vi "Kxx_Kxy_B_cs580_KEguard.vi"() -> ()   [LabVIEW 2023]
uses:
  Z:/Labview Control Software/Kxx_Kxy_B_cs580_v3_LV20/Z/Labview Control Software/Keithley 622x LV 2009/Utility/Typedefs/KE622x -- Instrument Type.ctl
  Typedefs/Kxx_Kxy_state_machine_cases.ctl
  Z:/Labview Control Software/Keithley 622x LV 2009/Typedefs/KE622x -- On Off Control.ctl
  Z:/Labview Control Software/Keithley 622x LV 2009/Configure/Output/Typedefs/KE6221 -- Output Response.ctl
  Z:/Labview Control Software/Keithley 622x LV 2009/Configure/Source/Typedefs/KE622x -- Voltage Limit.ctl
  <vilib>/Analysis/1siggen.llb/Ramp Pattern by Samples.vi
  <vilib>/Analysis/baseanly.llb/Mean (DBL).vi
  <vilib>/Instr/_visa.llb/VISA Configure Serial Port (Instr).vi
  <vilib>/Utility/file.llb/Read Delimited Spreadsheet (DBL).vi
  Global Variables/MQM Data Transfer All.vi
  <vilib>/Analysis/1siggen.llb/Ramp Pattern by Delta.vi
  <vilib>/Utility/file.llb/Write To Spreadsheet File (string).vi
  <instrlib>/Keithley 622x LV 2009/Keithley 622x.lvlib
  <vilib>/Analysis/NI_AALBase.lvlib
  Drivers/Keithley 2182/Keithley 2182.lvlib
  <vilib>/Analysis/NI_AALPro.lvlib
panel:
  out "error out":errorcluster
  in  "Kxy data":dbl[](array[numeric])
  in  "Kxx data":dbl[](array[numeric])
  in  "T_avg data":dbl[](array[numeric])
  in  "dTxx":dbl
  in  "HTR Power":dbl
  in  "dTxy":dbl
  in  "T_avg":dbl
  in  "T_H Array":dbl[](array[numeric])
  in  "T_C1 Array":dbl[](array[numeric])
  in  "T_C2 Array":dbl[](array[numeric])
  in  "HTR Voltage Array":dbl[](array[numeric])
  in  "?":enum32{"Setup", "Plotting", "Error Readouts"}(tab)
  in  "DeltaT (fraction of tsp)":dbl=0.05
  in  "Sample_t":dbl
  in  "Sample_w":dbl
  in  "Sample_Lxx":dbl
  in  "Heater Current File (H, T, current)":path
  out "Heater Current \nArray":dbl[](array[numeric])
  out "Ramp Pattern":dbl[](array[numeric])
  in  "Tstart (K)":dbl=3.0
  in  "Tend (K)":dbl=4.0
  in  "Steps":i16=2
  in  "Log (on)\nLin (off) (Temperature setpoints)":bool=TRUE
  in  "Initial Heater Current (A)":dbl=1e-06
  in  "Hstart (Oe)":dbl
  in  "Hend (Oe)":dbl
  in  "Field Steps":i16=1
  in  "Log (on)\nLin (off)  (Field setpoints)":bool
  in  "T_H Lockin":enum16{"LI1", "LI2", "LI3"}(ring)
  in  "T_C1 Lockin":enum16{"LI1", "LI2", "LI3"}(ring)=enum."LI2"
  in  "T_C2 Lockin":enum16{"LI1", "LI2", "LI3"}(ring)=enum."LI3"
  in  "Sample_Lxy":dbl=0.0005
  in  "Test?":bool
  in  "Calibration Only?":bool
  in  "Exchange gas?":bool
  in  "Preset Heater Current Array?":bool
  in  "T Current Source":refnum<visa-resource-name>="6221B"
  in  "HTR Current Source":refnum<visa-resource-name>="CS580-1"
  in  "DC Voltmeter":refnum<visa-resource-name>="2182"
  in  "Thermometer Frequency (Hz)":string="37"
  in  "Initial Thermometer Current (A)":string="1.4142e-7"
  in  "Final Field (Oe)":dbl
  in  "Final Temperature (K)":dbl=1.7
  in  "R_H coeffs file":path
  in  "R_C1 coeffs file":path
  in  "R_C2 coeffs file":path
  in  "R_C1 domain file":path
  in  "R_C2 domain file":path
  in  "R_H domain file":path
  in  "Field selection":u16(ring) items=["0.000000"]
  out "Calibration confirmed":bool
  out "R_C1 coeffs":dbl[](array[numeric])
  out "R_C2 coeffs":dbl[](array[numeric])
  out "R_H coeffs":dbl[](array[numeric])
  out "R_C1 Log Domain":dbl[](array[numeric])
  out "R_C2 Log Domain":dbl[](array[numeric])
  out "R_H Log Domain":dbl[](array[numeric])
  in  "Confirm Calibration":bool
  in  "Filename":path=path "C:/User Data/Luke/Kxx/NaYSe2/NaYSe2_1p7_100K_log_100_9T_8_23_21"
  in  "Heater Only?":bool
  in  "DC Keithley":refnum<visa-resource-name>
  out "Kxx Plot":cluster{dbl[], dbl[]}(graph)
  out "Kxy Plot":cluster{dbl[], dbl[]}(graph)
  out "All Data":cluster{dbl[], dbl[]}[](graph)
  in  "Finish":bool
  out "Data Rate (ms)":u32
  in  "Delay (ms)":dbl=300.0
  in  "Quick Data Recording":bool=TRUE
  out "Tsp":dbl
  out "HTR_Current":dbl
  out "Mask":dbl
  out "HTR_Voltage":dbl
  out "T_H":dbl
  out "T_C1":dbl
  out "I_therm":dbl
  out "T_C2":dbl
  in  "Display Elements":cluster{"X":bool, "Y":bool, "Name":u16}[](array[cluster]) {"Name" items=["Time (ms)", "Temperature (K)", "Field (T)", "LI_1_X", "LI_1_theta", "LI_3_X", "LI_3_theta", "LI_2_X", "LI_2_theta", "DC_V", "DC_I", "mask", "tsp", "I_therm", "T_H", "T_C1", "T_C2", "Fieldsp"]}
  in  "X-Axis":u16(ring) items=["Linear", "Reciprocal", "Log10"]
  in  "Y-Axis":u16(ring) items=["Linear", "Reciprocal", "Log10"]
  out "Fieldsp":dbl
  out "Global Stop":bool
  out "QD error out":errorcluster
  out "KE6221 error out":errorcluster
  out "KE2182 error out":errorcluster
  # "TURN ON HIGH VACUUM!"
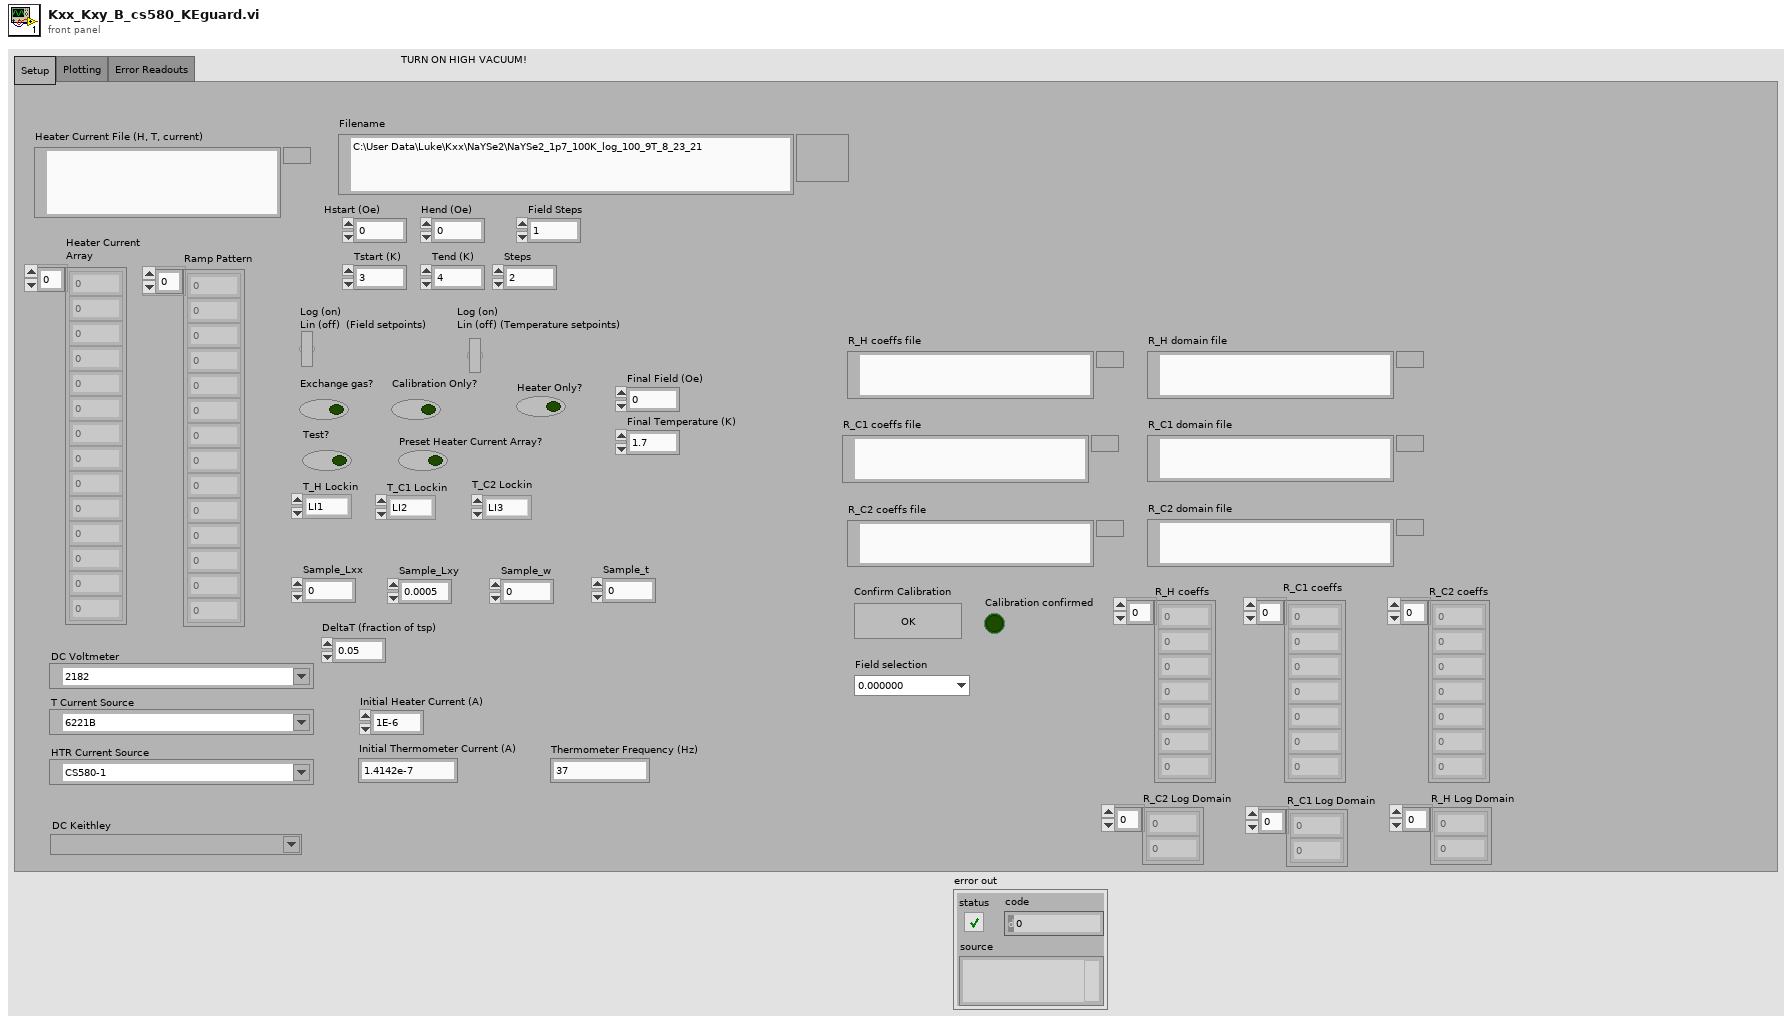
[diagram p1: front panel]
types:
  T1 = typedef "Keithley 622x.lvlib/KE622x -- Instrument Type.ctl" = enum16{"KE6220", "KE6221"}
  T2 = typedef "Kxx_Kxy_state_machine_cases.ctl" = enum16{"Initialize", "Wait to Stabilize (no heat)", "Measure (no heat)", "Turn on Heater, stabilize", "Measure (heat)", "Turn off Heater", "Assign Heater Current", "Plot Kxx, Kxy", "End"}
  T3 = typedef "Keithley 622x.lvlib/KE622x -- Voltage Limit.ctl" = dbl
  T4 = typedef "Keithley 622x.lvlib/KE6221 -- Output Response.ctl" = enum16{"Fast", "Slow"}
  T5 = typedef "Keithley 622x.lvlib/KE622x -- On Off Control.ctl" = enum16{"Off", "On"}
  T6 = cluster{"T_avg data":dbl[], "Kxx data":dbl[], "Kxy data":dbl[]}
  T7 = cluster{"T_avg":dbl, "dTxx":dbl, "dTxy":dbl, "HTR Power":dbl, "HTR Voltage Array":dbl[], "T_H Array":dbl[], "T_C1 Array":dbl[], "T_C2 Array":dbl[], "error out":errorcluster}
  T8 = typedef "ZI_Frontpanel_All.ctl" = cluster{"Lockin 1 Demod 0":cluster{"R(V)":dbl, "Theta (deg)":dbl, "Timestamp (ms)":u32, "X(V)":dbl, "Y(V)":dbl, "frequency (Hz)":dbl, "output voltage (V)":dbl}, "Lockin 2 Demod 0":cluster{"R(V)":dbl, "Theta (deg)":dbl, "Timestamp (ms)":u32, "X(V)":dbl, "Y(V)":dbl, "frequency (Hz)":dbl, "output voltage (V)":dbl}, "Lockin 3 Demod 0":cluster{"R(V)":dbl, "Theta (deg)":dbl, "Timestamp (ms)":u32, "X(V)":dbl, "Y(V)":dbl, "frequency (Hz)":dbl, "output voltage (V)":dbl}, "Lockin 4 Demod 0":cluster{"R(V)":dbl, "Theta (deg)":dbl, "Timestamp (ms)":u32, "X(V)":dbl, "Y(V)":dbl, "frequency (Hz)":dbl, "output voltage (V)":dbl}, "LI1 active":bool, "LI2 active":bool, "LI3 active":bool, "LI4 active":bool}
  T9 = typedef "PPMS_Status.ctl" = cluster{"Field":cluster{"Field (T)":dbl, "Field stable":bool, "Timestamp (ms)":u32}, "Temperature":cluster{"Temperature (K)":dbl, "Temperature stable":bool, "Timestamp (ms)":u32}}
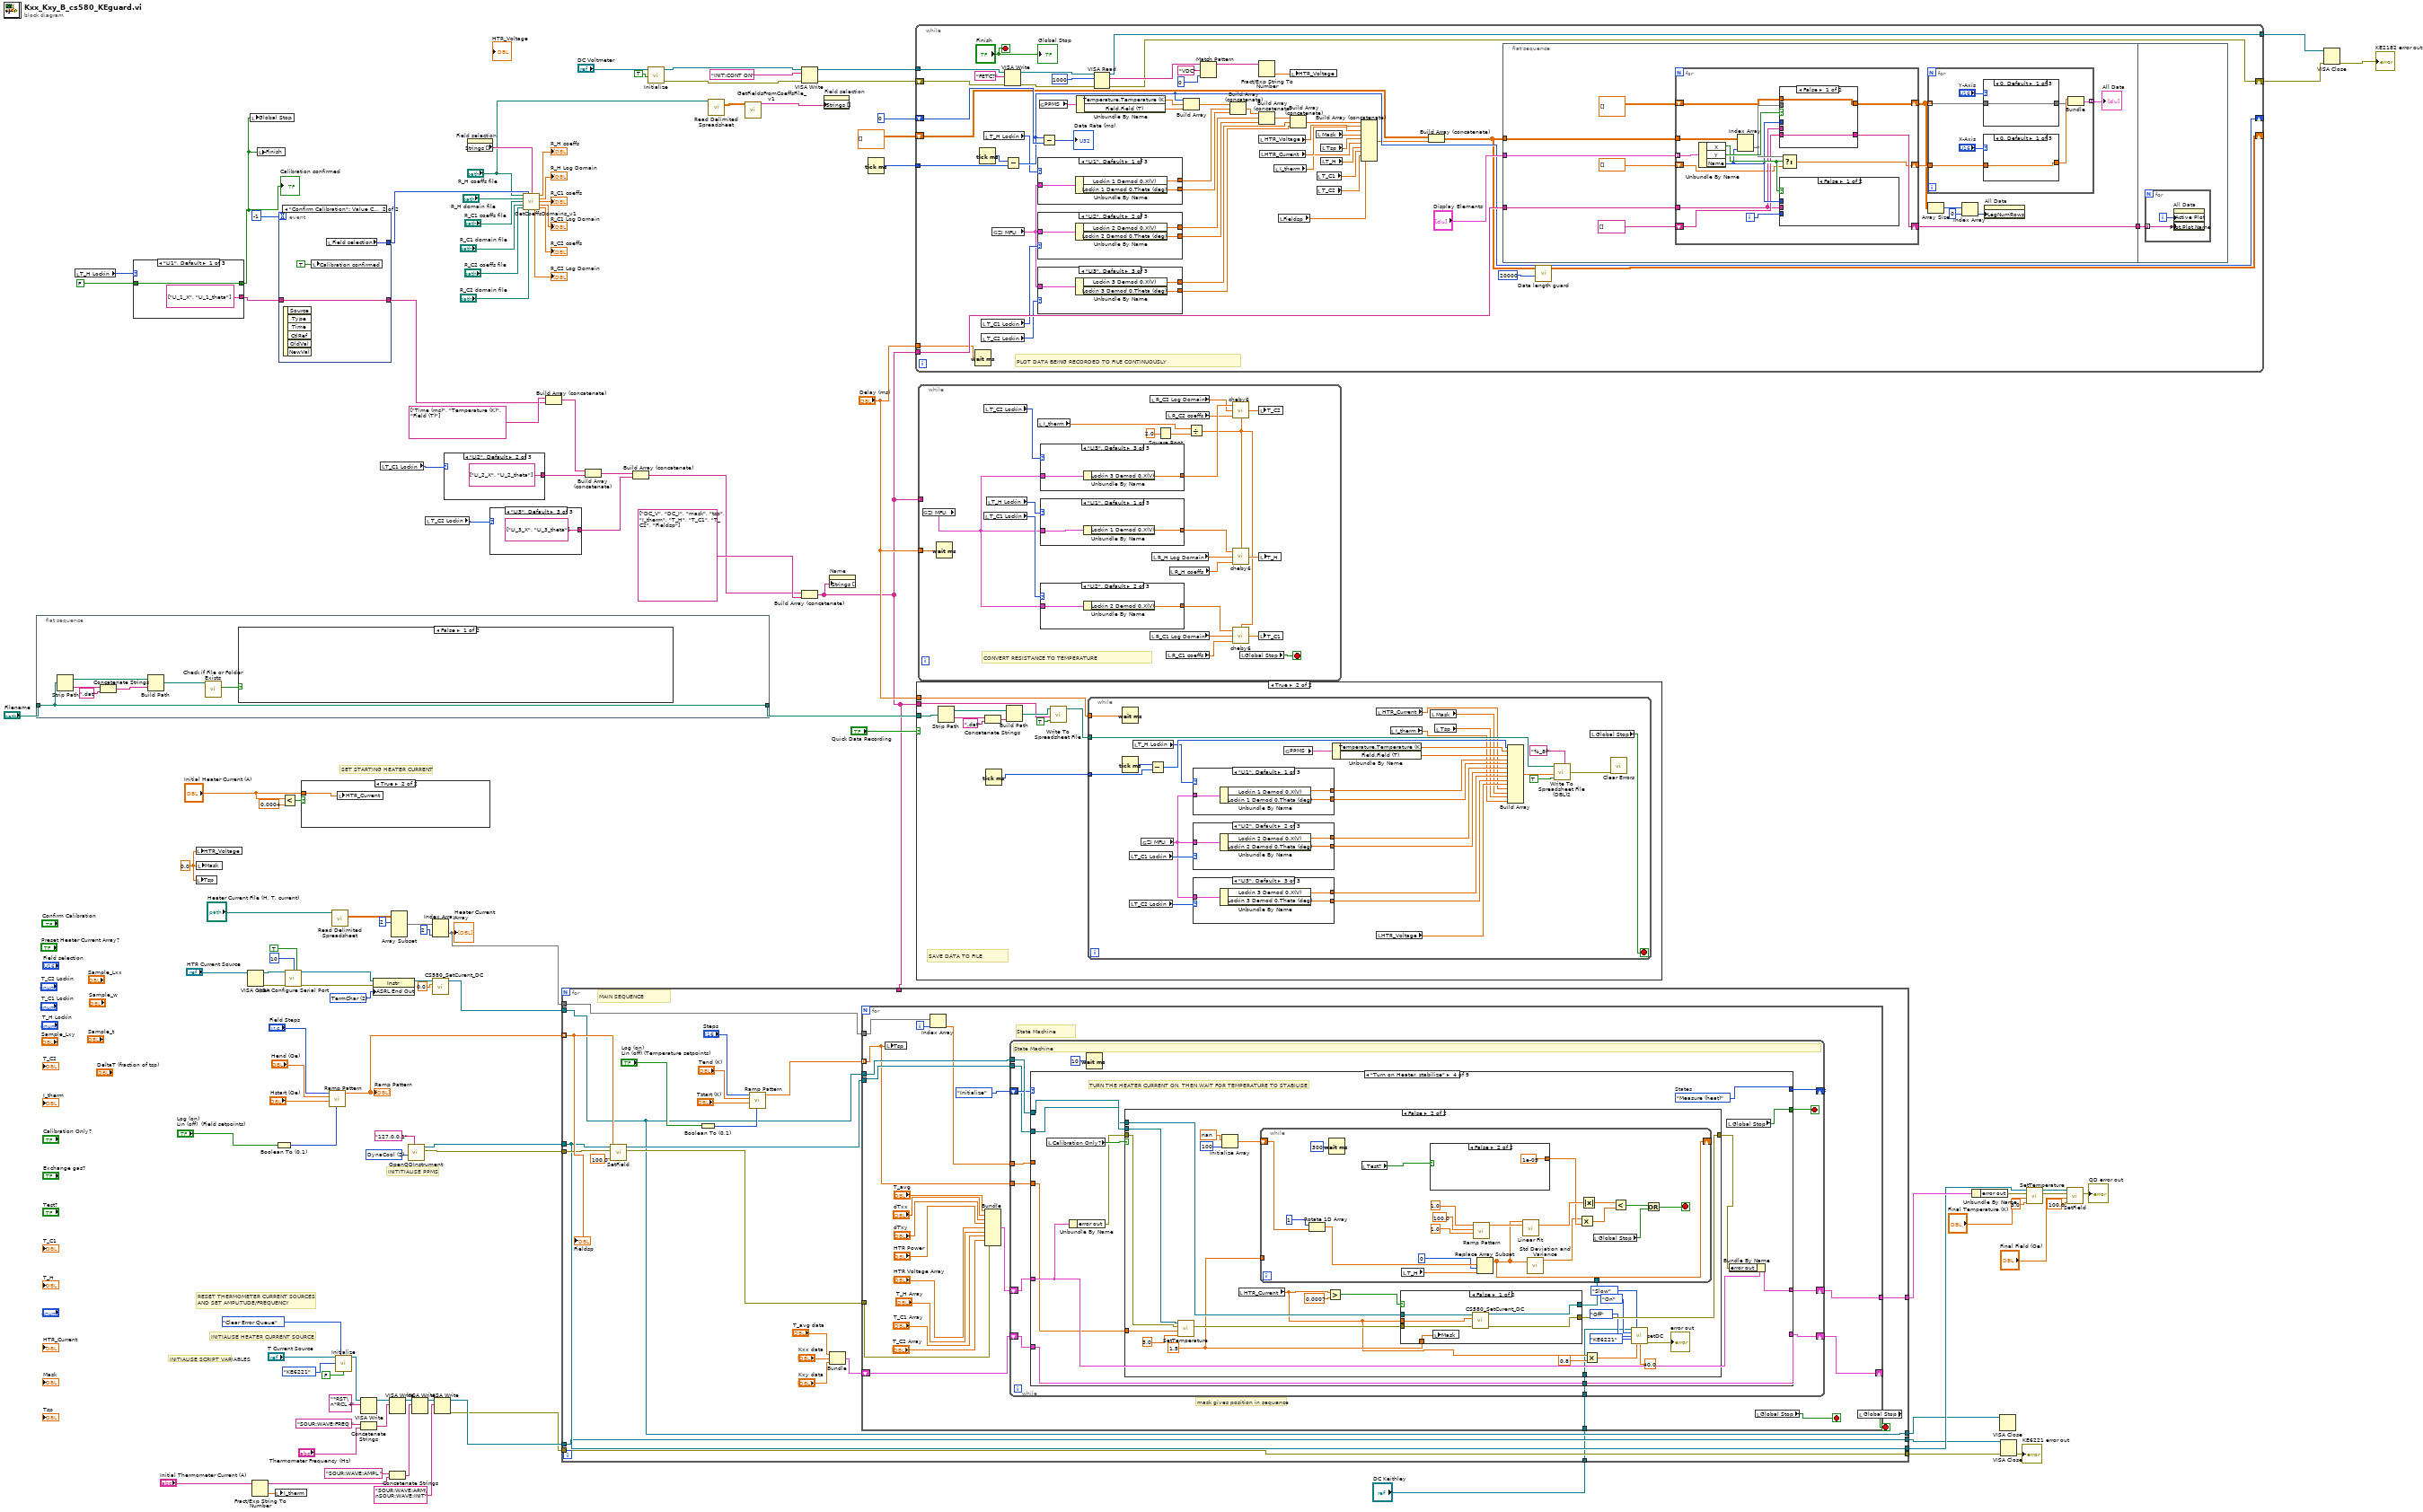
[diagram p0: block diagram]
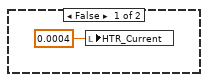
[diagram p2: hidden frame]
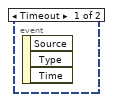
[diagram p3: hidden frame]
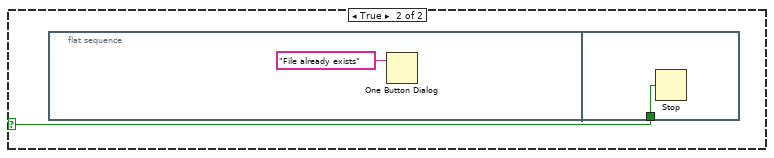
[diagram p4: hidden frame]
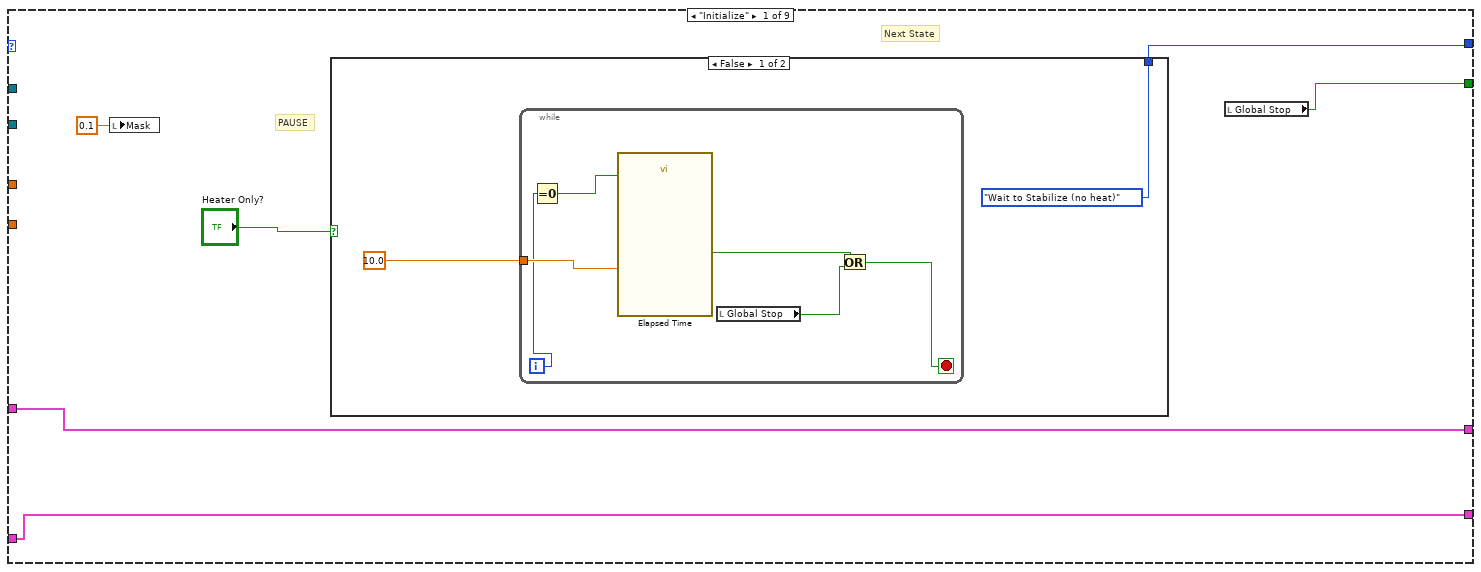
[diagram p5: hidden frame]
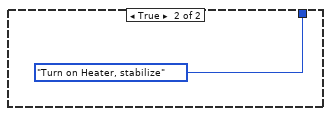
[diagram p6: hidden frame]
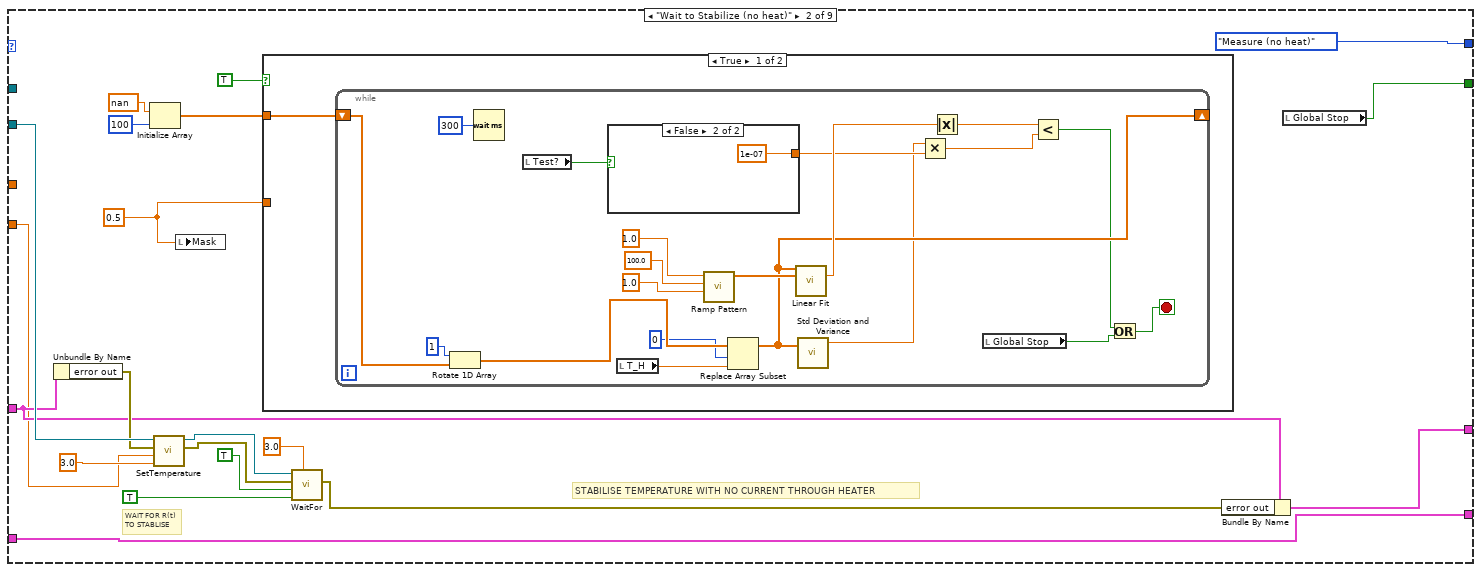
[diagram p7: hidden frame]
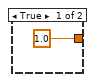
[diagram p8: hidden frame]
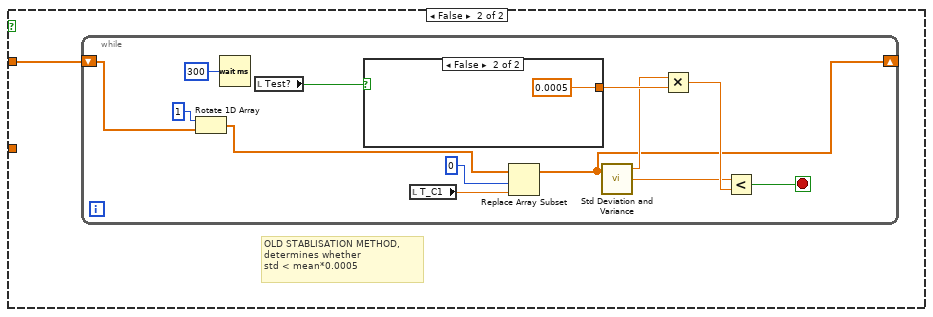
[diagram p9: hidden frame]
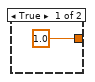
[diagram p10: hidden frame]
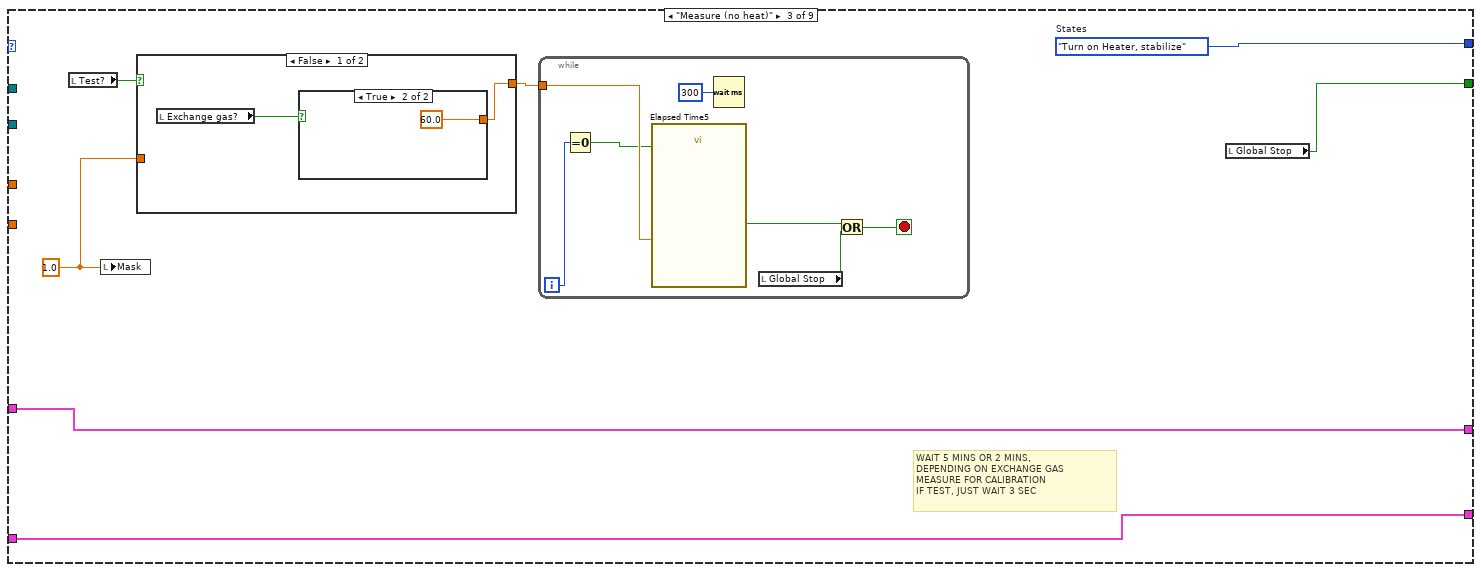
[diagram p11: hidden frame]
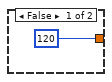
[diagram p12: hidden frame]
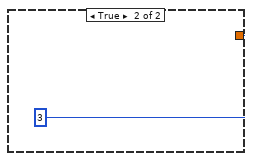
[diagram p13: hidden frame]
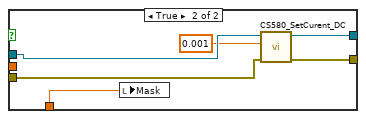
[diagram p15: hidden frame]
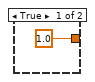
[diagram p16: hidden frame]
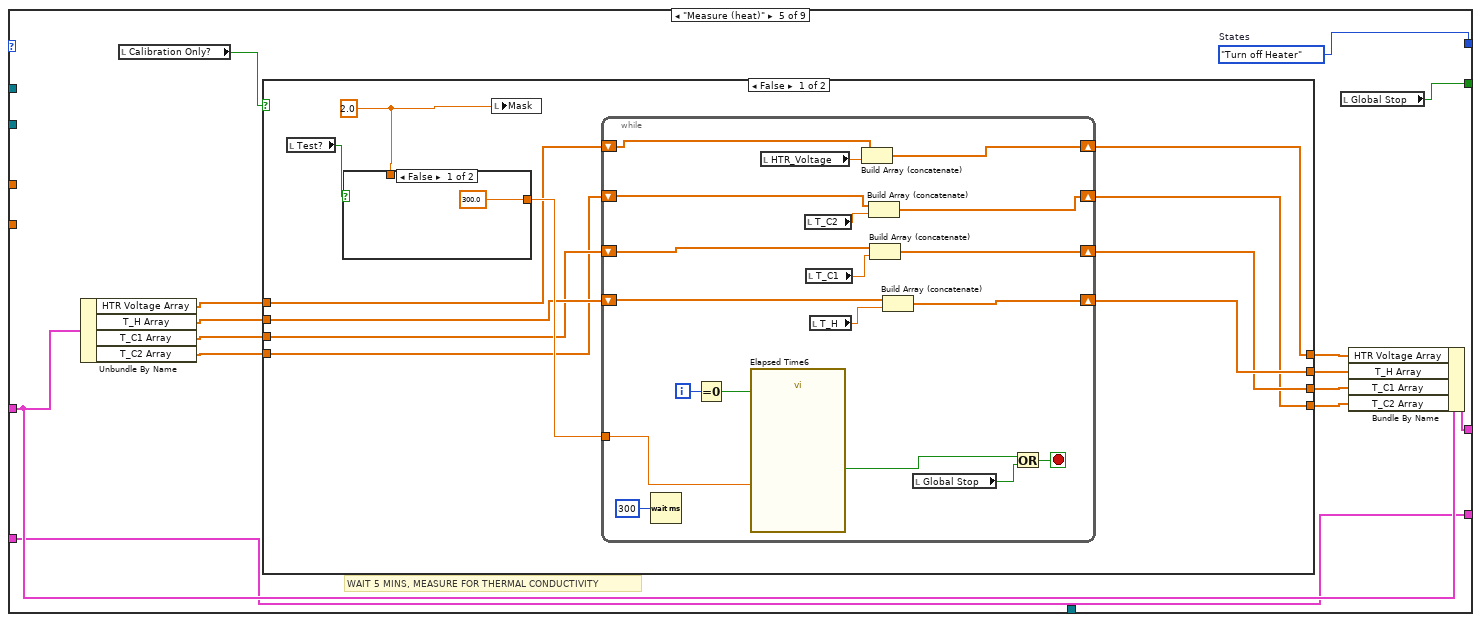
[diagram p17: hidden frame]
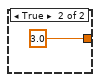
[diagram p18: hidden frame]
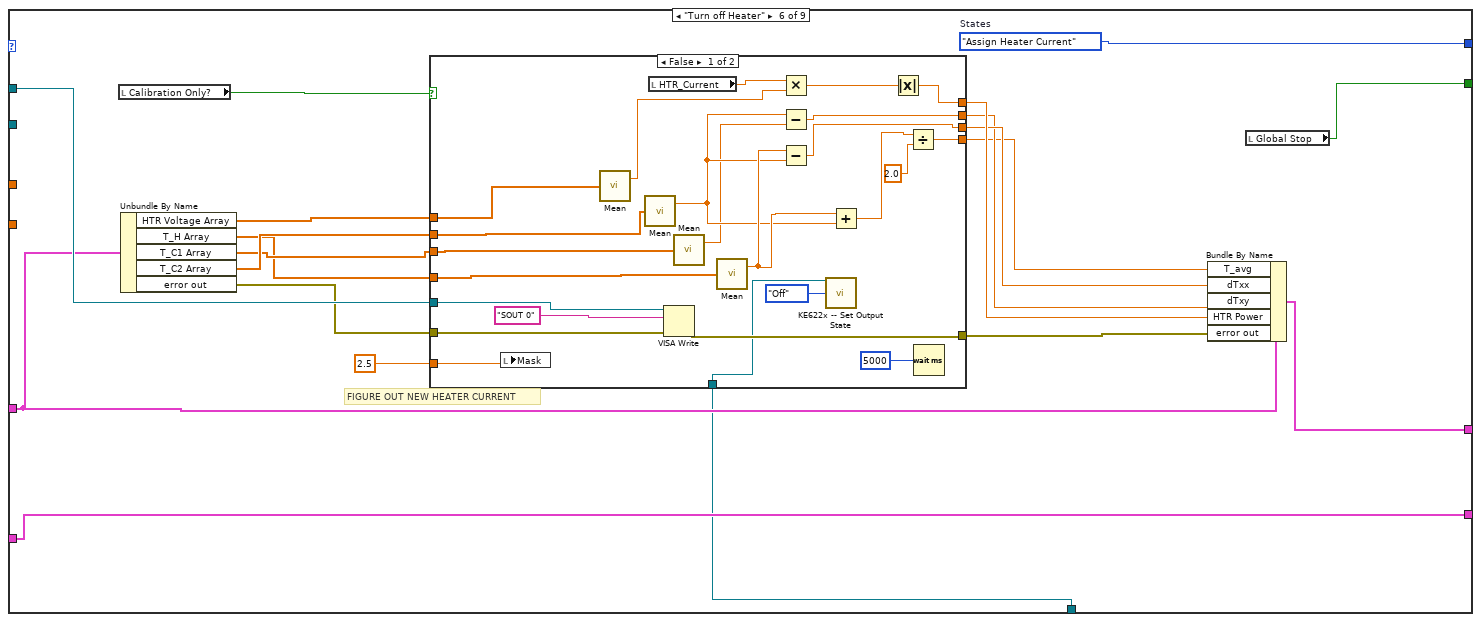
[diagram p20: hidden frame]
diagram:
  w85 = u16 2 items=["None", "Last Bit", "TermChar", "Break"] ("Serial Settings:End Mode for Writes")
  w103 = 0.0 ("Mask")
  w110 = 2 items=["PPMS", "VersaLab", "DynaCool", "SVSM"] ("Instrument Type")
  # "SET STARTING HEATER CURRENT"
  # "INITIALISE HEATER CURRENT SOURCE"
  # "RESET THERMOMETER CURRENT SOURCES\nAND SET AMPLITUDE/FREQUENCY"
  # "INITITIALISE PPMS"
  # "INITIALISE SCRIPT VARIABLES"
  n1 = flat-sequence {
    tunnel: "Filename" -> [w117]
    tunnel: [w117] -> w37
    frame #0 {
      n2 = Strip Path(path=w117) -> (stripped path=w121:path, name=w118:string)
      n3 = Concatenate Strings(w118, ".dat") -> (w120:string)
      n4 = Build Path(base path=w121, name or relative path=w120) -> (appended path=w116:path)
      n5 = call <vilib>:"Check if File or Folder Exists.vi"("path"=w116) -> ("file or folder exists?"=w115:bool)  [unwired: 8 in, 2 out]
      n6 = case shown="False" w115 {
        selector: w115 -> [_ w122]
        frame False {
        }
        frame True {
          n7 = flat-sequence {
            tunnel: w122 -> [w124]
            frame #0 {
              n8 = One Button Dialog(message="File already exists") -> ()  [unwired: 1 in, 1 out]
            }
            frame #1 {
              n9 = Stop(stop? (T)=w124) -> ()
            }
          }
        }
      }
    }
  }
  n10 = local read "T_H Lockin"() -> (w78:enum16{"LI1", "LI2", "LI3"})
  n11 = case shown="\"LI1\", Default" w78 {
    tunnel: [string[] ["LI_1_X", "LI_1_theta"] ("element") string[] ["LI_2_X", "LI_2_theta"] ("element") string[] ["LI_3_X", "LI_3_theta"] ("element")] -> w35
    tunnel: FALSE ("Calibration confirmed") -> [w125 w127 w129]
    tunnel: [w125 w127 w129] -> w2
    frame "LI1", Default {
    }
    frame "LI2" {
    }
    frame "LI3" {
    }
  }
  "Calibration confirmed" <- w2
  n12 = local write "HTR_Voltage"(w103) -> ()
  n13 = local write "Tsp"(w103) -> ()
  n14 = local write "Mask"(w103) -> ()
  n15 = VISA Open(VISA resource name="HTR Current Source") -> (VISA resource name=w81:refnum<visa-resource-name>, error out=w82:errorcluster)  [unwired: 4 in]
  n16 = local write "Global Stop"(w2) -> ()
  n17 = Fract/Exp String To Number(string="Initial Thermometer Current (A)") -> (number=w93:dbl)  [unwired: 3 in, 1 out]
  n18 = local write "Finish"(w2) -> ()
  n19 = local write "I_therm"(w93) -> ()
  n20 = Boolean To (0,1)(Boolean="Log (on)\nLin (off)  (Field setpoints)") -> (0, 1=w88:i16)
  n21 = event shown="[1] \"Confirm Calibration\": Value Change" {
    selector: _ -> [_ _]
    dyn-events: _ -> [_ _]
    timeout: -1 -> [_ _]
    tunnel: w35 -> [_ w133]
    tunnel: [_ w133] -> w34
    tunnel: [_ w131] -> w32
    event Timeout {
      n22 = event-data() -> ()  [unwired: 1 in, 3 out]
    }
    event "Confirm Calibration": Value Change {
      n23 = event-data() -> ()  [unwired: 1 in, 6 out]
      n24 = local write "Calibration confirmed"(TRUE ("Calibration confirmed")) -> ()
      n25 = local read "Field selection"() -> (w131:u16)
    }
  }
  n26 = Less?(x="Initial Heater Current (A)", y=0.0004) -> (x < y?=w28:bool)
  n27 = call-poly "VISA Configure Serial Port"("VISA resource name"=w81, "termination char\n(0xA = '\\n' = LF)"=u8 10 ("termination char\n(0xA = '\\n' = LF)"), "Enable Termination\nChar (T)"=TRUE ("Enable Termination\nChar (T)"), "error in (no error)"=w82) -> ("VISA resource name out"=w83:refnum<visa-resource-name>, "error out"=w84:errorcluster)  [unwired: 10 in]
  n28 = case shown="True" w28 {
    tunnel: "Initial Heater Current (A)" -> [_ w135]
    frame False {
      n29 = local write "HTR_Current"(0.0004 ("HTR_Current")) -> ()
    }
    frame True {
      n30 = local write "HTR_Current"(w135) -> ()
    }
  }
  n31 = call-poly <vilib>:"Ramp Pattern.vi"("type"=w88, "start"="Hstart (Oe)", "end"="Hend (Oe)", "samples"="Field Steps") -> ("Ramp Pattern"=w56:dbl[])  [unwired: 6 in, 1 out]
  "Ramp Pattern" <- w56
  n32 = call-poly <vilib>:"Read Delimited Spreadsheet.vi"("file path (dialog if empty)"="Heater Current File (H, T, current)") -> ("all rows"=w66:dbl[][])  [unwired: 9 in, 5 out]
  n33 = call "Initialize.vi"("VISA resource name"="T Current Source", "Error Queue Option"=enum16{"Clear Error Queue", "Error Query"}."Clear Error Queue", "Instrument Type"=KE622x_--_Instrument_Type."KE6221", "Reset? (T)"=FALSE) -> ("VISA resource name out"=w101:refnum<visa-resource-name>)  [unwired: 10 in, 1 out]
  n34 = VISA Write(VISA resource name=w101, write buffer="*RST\n*RCL 4") -> (VISA resource name out=w95:refnum<visa-resource-name>)  [unwired: 1 in, 2 out]
  n35 = Concatenate Strings("SOUR:WAVE:FREQ " ("string"), "Thermometer Frequency (Hz)") -> (w100:string)
  n36 = property class="Instr"(reference=w83, error in=w84, "ASRL End Out"=w85) -> (reference out=w69:refnum<visa-resource-name>)  [unwired: 1 out]
  n37 = local read "T_C1 Lockin"() -> (w77:enum16{"LI1", "LI2", "LI3"})
  n38 = VISA Write(VISA resource name=w95, write buffer=w100) -> (VISA resource name out=w94:refnum<visa-resource-name>)  [unwired: 1 in, 2 out]
  n39 = Concatenate Strings("SOUR:WAVE:AMPL " ("string"), "Initial Thermometer Current (A)") -> (w97:string)
  n40 = Array Subset(array=w66, index (row)=2 ("index")) -> (w64:dbl[][])  [unwired: 3 in]
  n41 = call <instrlib>:"OpenQDInstrument.vi"("IP Address"="127.0.0.1", "Instrument Type"=w110) -> ("error out"=w31:errorcluster, "Instrument Ref"=w29:refnum<k24>)  [unwired: 6 in]
  n42 = VISA Write(VISA resource name=w94, write buffer=w97) -> (VISA resource name out=w57:refnum<visa-resource-name>)  [unwired: 1 in, 2 out]
  n43 = local read "T_C2 Lockin"() -> (w73:enum16{"LI1", "LI2", "LI3"})
  n44 = Index Array(array=w64, index (col)=2 ("disabled index (col)")) -> (element=w55:dbl[])  [unwired: 1 in]
  "Heater Current \nArray" <- w55
  n45 = call "CS580_SetCurent_DC.vi"("Current (A)"=0.0, "VISA Refnum in"=w69) -> ("VISA resource name out"=w30:refnum<visa-resource-name>)  [unwired: 8 in, 1 out]
  n46 = VISA Write(VISA resource name=w57, write buffer="SOUR:WAVE:ARM\nSOUR:WAVE:INIT") -> (VISA resource name out=w22:refnum<visa-resource-name>, error out=w18:errorcluster)  [unwired: 1 in, 1 out]
  n47 = case shown="\"LI2\", Default" w77 {
    tunnel: [string[] ["LI_1_X", "LI_1_theta"] ("element") string[] ["LI_2_X", "LI_2_theta"] ("element") string[] ["LI_3_X", "LI_3_theta"] ("element")] -> w75
    frame "LI1" {
    }
    frame "LI2", Default {
    }
    frame "LI3" {
    }
  }
  n48 = property on="Field selection" class="Ring (strict)"() -> ("Strings []"=w47:string[])  [unwired: 2 in, 2 out]
  n49 = case shown="\"LI3\", Default" w73 {
    tunnel: [string[] ["LI_1_X", "LI_1_theta"] ("element") string[] ["LI_2_X", "LI_2_theta"] ("element") string[] ["LI_3_X", "LI_3_theta"] ("element")] -> w71
    frame "LI1" {
    }
    frame "LI2" {
    }
    frame "LI3", Default {
    }
  }
  n50 = call "GetCoeffsDomains_v1.vi"("R_H coeffs file"="R_H coeffs file", "Field index"=w32, "Fields"=w47, "R_H domain file"="R_H domain file", "R_C1 coeffs file"="R_C1 coeffs file", "R_C1 domain file"="R_C1 domain file", "R_C2 coeffs file"="R_C2 coeffs file", "R_C2 domain file"="R_C2 domain file") -> ("R_H coeffs"=→"R_H coeffs":dbl[], "R_H Log Domain"=→"R_H Log Domain":dbl[], "R_C1 coeffs"=→"R_C1 coeffs":dbl[], "R_C1 Log Domain"=→"R_C1 Log Domain":dbl[], "R_C2 Log Domain"=→"R_C2 Log Domain":dbl[], "R_C2 coeffs"=→"R_C2 coeffs":dbl[])  [unwired: 2 in]
  n51 = Build Array (concatenate)(string[] ["Time (ms)", "Temperature (K)", "Field (T)"], w34) -> (w76:string[])
  n52 = Build Array (concatenate)(w76, w75) -> (w72:string[])
  n53 = Build Array (concatenate)(w72, w71) -> (w70:string[])
  n54 = call "Initialize.vi"("Reset (True)"=TRUE, "VISA resource name"="DC Voltmeter") -> ("error out"=w106:errorcluster, "VISA resource name out"=w105:refnum<visa-resource-name>)  [unwired: 8 in]
  n55 = call-poly <vilib>:"Read Delimited Spreadsheet.vi"("file path (dialog if empty)"="R_H coeffs file") -> ("all rows"=w12:dbl[][])  [unwired: 9 in, 5 out]
  n56 = call "GetFieldsFromCoeffsFile_v1.vi"("all rows"=w12) -> ("Array"=w62:string[])  [unwired: 10 in]
  n57 = VISA Write(VISA resource name=w105, write buffer="INIT:CONT ON", error in (no error)=w106) -> (VISA resource name out=w50:refnum<visa-resource-name>, error out=w49:errorcluster)  [unwired: 1 out]
  n58 = Build Array (concatenate)(w70, string[] ["DC_V", "DC_I", "mask", "tsp", "I_therm", "T_H", "T_C1", "T_C2", "Fieldsp"] ("element")) -> (w3:string[])
  n59 = for {
    tunnel: w56 -> [w164] mode=indexing
    tunnel: w29 -> [w147]
    tunnel: w31 -> [w162]
    tunnel: w55 -> [w155]
    tunnel: w30 -> [w143]
    tunnel: [w148] -> w24
    tunnel: w22 -> [w146]
    tunnel: [w147] -> w21
    tunnel: [w146] -> w20
    tunnel: w18 -> [w145]
    tunnel: [w145] -> w17
    tunnel: [w143] -> w4
    tunnel: w3 -> [_]
    tunnel: "DC Keithley" -> [w142]
    stop <- w144 stop-if-true
    # "MAIN SEQUENCE"
    n60 = call <instrlib>:"SetField.vi"("Rate"=100.0, "Field"=w164, "error in (no error)"=w162, "Instrument Ref In"=w147) -> ("error out"=w154:errorcluster, "Instrument Ref Out"=w153:refnum<k24>)  [unwired: 3 in, 1 out]
    n61 = Boolean To (0,1)(Boolean="Log (on)\nLin (off) (Temperature setpoints)") -> (0, 1=w159:i16)
    n62 = call-poly <vilib>:"Ramp Pattern.vi"("type"=w159, "start"="Tstart (K)", "end"="Tend (K)", "samples"="Steps") -> ("Ramp Pattern"=w161:dbl[])  [unwired: 6 in, 1 out]
    n63 = Bundle("T_avg data"="T_avg data", "Kxx data"="Kxx data", "Kxy data"="Kxy data") -> (w149:T6)  [unwired: 1 in]
    n64 = for {
      tunnel: w161 -> [w168] mode=indexing
      tunnel: w155 -> [w186]
      tunnel: w154 -> [w173]
      tunnel: w143 -> [w183]
      tunnel: w153 -> [w182]
      shift-right: [w167] -> _
      shift-left: w149 -> [w166]
      tunnel: [w170] -> w148
      tunnel: w142 -> [w165]
      i -> [w185]
      stop <- w169 stop-if-true
      # "State Machine"
      # "mask gives position in sequence"
      n65 = local write "Tsp"(w168) -> ()
      n66 = Index Array(array=w186, index=w185) -> (element=w171:dbl)
      n67 = Bundle("T_avg"="T_avg", "dTxx"="dTxx", "dTxy"="dTxy", "HTR Power"="HTR Power", "HTR Voltage Array"="HTR Voltage Array", "T_H Array"="T_H Array", "T_C1 Array"="T_C1 Array", "T_C2 Array"="T_C2 Array", "error out"=w173) -> (w172:T7)  [unwired: 1 in]
      n68 = while {
        shift-right: [w199] -> _
        shift-left: Kxx_Kxy_state_machine_cases."Initialize" -> [w196]
        tunnel: w183 -> [w197]
        tunnel: w182 -> [w192]
        shift-right: [w195] -> w170
        shift-left: w172 -> [w194]
        tunnel: w171 -> [w193]
        tunnel: w168 -> [w190]
        shift-right: [w189] -> w167
        shift-left: w166 -> [w188]
        tunnel: w165 -> [w187]
        stop <- w191 stop-if-true
        # "State Machine"
        n69 = case shown="\"Turn on Heater, stabilize\"" w196 {
          selector: w196 -> [_ _ _ _ _ _ _ _ w534]
          tunnel: w192 -> [_ w225 _ w303 _ _ _ _ _]
          tunnel: [w204 Kxx_Kxy_state_machine_cases."Measure (no heat)" w278 w301 w376 w430 w484 w522 w534] -> w199
          tunnel: w197 -> [_ _ _ w302 _ w431 _ _ _]
          tunnel: [w203 w220 w277 w297 w367 w418 w482 w521 w533] -> w195
          tunnel: w194 -> [w203 w222 w277 w299 w366 w425 w482 w521 w533]
          tunnel: w188 -> [w202 w219 w276 w296 w365 w417 w481 w512 w532]
          tunnel: [w202 w219 w276 w296 w365 w417 w481 w508 w532] -> w189
          tunnel: w193 -> [_ _ _ _ _ _ w480 _ _]
          tunnel: [w201 w218 w275 w295 w364 w416 w479 w505 TRUE] -> w191
          tunnel: w190 -> [_ w215 _ w294 _ _ _ _ _]
          tunnel: w187 -> [_ _ _ w293 _ w414 _ _ _]
          frame "Initialize" {
            # "Next State"
            # "PAUSE"
            n70 = local write "Mask"(0.1 ("Mask")) -> ()
            n71 = case shown="False" "Heater Only?" {
              tunnel: [Kxx_Kxy_state_machine_cases."Wait to Stabilize (no heat)" Kxx_Kxy_state_machine_cases."Turn on Heater, stabilize"] -> w204
              frame False {
                n72 = while {
                  tunnel: 10.0 ("Time Target (s)") -> [w213]
                  i -> [w209]
                  stop <- w210 stop-if-true
                  n73 = Equal To 0?(x=w209) -> (x = 0?=w208:bool)
                  n74 = call "Elapsed Time"("Time Target (s)"=w213, "Reset"=w208) -> ("Time has Elapsed"=w212:bool)  [unwired: 10 in, 7 out]
                  n75 = local read "Global Stop"() -> (w211:bool)
                  n76 = Or(x=w212, y=w211) -> (x .or. y?=w210:bool)
                }
              }
              frame True {
              }
            }
            n77 = local read "Global Stop"() -> (w201:bool)
          }
          frame "Wait to Stabilize (no heat)" {
            w216 = 0.5 ("Mask")
            # "STABILISE TEMPERATURE WITH NO CURRENT THROUGH HEATER"
            # "WAIT FOR R(t)\nTO STABLISE"
            n78 = Unbundle By Name(w222) -> ("error out"=w223:errorcluster)
            n79 = Initialize Array(nan ("Element"), 100) -> (w233:dbl[])
            n80 = call <instrlib>:"SetTemperature.vi"("Rate"=3.0, "Temperature"=w215, "error in (no error)"=w223, "Instrument Ref In"=w225) -> ("error out"=w234:errorcluster, "Instrument Ref Out"=w217:refnum<k24>)  [unwired: 3 in, 1 out]
            n81 = local write "Mask"(w216) -> ()
            n82 = case shown="True" TRUE {
              tunnel: w233 -> [w235 w258]
              tunnel: w216 -> [_ _]
              frame True {
                n83 = while {
                  shift-right: [w243] -> _
                  shift-left: w235 -> [w252]
                  stop <- w236 stop-if-true
                  n84 = Rotate 1D Array(1:w252, 2:1 ("n")) -> (0:w255:dbl[])
                  n85 = Wait (ms)(milliseconds to wait=u32 300) -> ()  [unwired: 1 out]
                  n86 = local read "Test?"() -> (w239:bool)
                  n87 = case shown="False" w239 {
                    tunnel: [1.0 ("y") 1e-07 ("y")] -> w242
                    frame True {
                    }
                    frame False {
                    }
                  }
                  n88 = local read "T_H"() -> (w251:dbl)
                  n89 = call-poly <vilib>:"Ramp Pattern.vi"("start"=1.0, "end"=100.0, "delta"=1.0) -> ("Ramp Pattern"=w247:dbl[])  [unwired: 6 in, 2 out]
                  n90 = Replace Array Subset(array=w255, new element=w251, index=0 ("Index")) -> (w243:dbl[])
                  n91 = call <vilib>:"Linear Fit.vi"("Y"=w243, "X"=w247) -> ("slope"=w245:dbl)  [unwired: 9 in, 4 out]
                  n92 = call <vilib>:"Std Deviation and Variance.vi"("X"=w243) -> ("mean"=w240:dbl)  [unwired: 1 in, 2 out]
                  n93 = Multiply(x=w240, y=w242) -> (x*y=w241:dbl)
                  n94 = Absolute Value(x=w245) -> (abs(x)=w244:dbl)
                  n95 = local read "Global Stop"() -> (w238:bool)
                  n96 = Less?(x=w244, y=w241) -> (x < y?=w237:bool)
                  n97 = Or(x=w237, y=w238) -> (x .or. y?=w236:bool)
                }
              }
              frame False {
                # "OLD STABLISATION METHOD,\ndetermines whether \nstd < mean*0.0005"
                n98 = while {
                  shift-right: [w261] -> _
                  shift-left: w258 -> [w267]
                  stop <- w262 stop-if-true
                  n99 = Rotate 1D Array(1:w267, 2:1 ("n")) -> (0:w270:dbl[])
                  n100 = Wait (ms)(milliseconds to wait=u32 300) -> ()  [unwired: 1 out]
                  n101 = local read "Test?"() -> (w259:bool)
                  n102 = case shown="False" w259 {
                    tunnel: [1.0 ("y") 0.0005 ("y")] -> w265
                    frame True {
                    }
                    frame False {
                    }
                  }
                  n103 = local read "T_C1"() -> (w260:dbl)
                  n104 = Replace Array Subset(array=w270, new element=w260, index=0 ("Index")) -> (w261:dbl[])
                  n105 = call <vilib>:"Std Deviation and Variance.vi"("X"=w261) -> ("mean"=w264:dbl, "standard deviation"=w263:dbl)  [unwired: 1 in, 1 out]
                  n106 = Multiply(x=w264, y=w265) -> (x*y=w266:dbl)
                  n107 = Less?(x=w263, y=w266) -> (x < y?=w262:bool)
                }
              }
            }
            n108 = call <instrlib>:"WaitFor.vi"("Delay"=3.0, "Wait For Field"=TRUE, "Wait For Temperature"=TRUE, "error in (no error)"=w234, "Instrument Ref In"=w217) -> ("error out"=w221:errorcluster)  [unwired: 5 in, 1 out]
            n109 = Bundle By Name(cluster=w222, "error out"=w221) -> (w220:T7)
            n110 = local read "Global Stop"() -> (w218:bool)
          }
          frame "Measure (no heat)" {
            w278 = Kxx_Kxy_state_machine_cases."Turn on Heater, stabilize"  # States
            w274 = 1.0 ("Mask")
            # "WAIT 5 MINS OR 2 MINS, \nDEPENDING ON EXCHANGE GAS\nMEASURE FOR CALIBRATION\nIF TEST, JUST WAIT 3 SEC"
            n111 = local read "Test?"() -> (w280:bool)
            n112 = local write "Mask"(w274) -> ()
            n113 = case shown="False" w280 {
              tunnel: [w281 u32 3 ("milliseconds to wait")] -> w279
              tunnel: w274 -> [_ _]
              frame False {
                n114 = local read "Exchange gas?"() -> (w282:bool)
                n115 = case shown="True" w282 {
                  tunnel: [120 60.0 ("Time to Wait (s)")] -> w281
                  frame False {
                  }
                  frame True {
                  }
                }
              }
              frame True {
              }
            }
            n116 = while {
              tunnel: w279 -> [w290]
              i -> [w287]
              stop <- w289 stop-if-true
              n117 = Equal To 0?(x=w287) -> (x = 0?=w286:bool)
              n118 = call "Elapsed Time5"("Time Target (s)"=w290, "Reset"=w286) -> ("Time has Elapsed"=w288:bool)  [unwired: 10 in, 7 out]
              n119 = Wait (ms)(milliseconds to wait=u32 300) -> ()  [unwired: 1 out]
              n120 = local read "Global Stop"() -> (w292:bool)
              n121 = Or(x=w288, y=w292) -> (x .or. y?=w289:bool)
            }
            n122 = local read "Global Stop"() -> (w275:bool)
          }
          frame "Turn on Heater, stabilize" {
            w301 = Kxx_Kxy_state_machine_cases."Measure (heat)"  # States
            # "TURN THE HEATER CURRENT ON, THEN WAIT FOR TEMPERATURE TO STABILISE"
            n123 = local read "Calibration Only?"() -> (w304:bool)
            n124 = Unbundle By Name(w299) -> ("error out"=w300:errorcluster)
            n125 = case shown="False" w304 {
              tunnel: w303 -> [_ w329]
              tunnel: w300 -> [w305 w321]
              tunnel: [w305 w322] -> w298
              tunnel: w302 -> [_ w323]
              tunnel: w294 -> [_ w317]
              tunnel: w293 -> [_ w307]
              frame True {
              }
              frame False {
                w319 = 1.5 ("Mask")
                n126 = call <instrlib>:"SetTemperature.vi"("Rate"=3.0, "Temperature"=w317, "error in (no error)"=w321, "Instrument Ref In"=w329) -> ("error out"=w320:errorcluster)  [unwired: 3 in, 2 out]
                n127 = Initialize Array(nan ("Element"), 100) -> (w328:dbl[])
                n128 = local read "HTR_Current"() -> (w310:dbl)
                n129 = Greater?(x=w310, y=0.0007) -> (0:w324:bool)
                n130 = case shown="False" w324 {
                  tunnel: w320 -> [w333 w341]
                  tunnel: w323 -> [w334 w340]
                  tunnel: [w331 w339] -> w322
                  tunnel: [w332 w338] -> w318
                  tunnel: w310 -> [w335 _]
                  tunnel: w319 -> [w330 w336]
                  frame False {
                    n131 = local write "Mask"(w330) -> ()
                    n132 = call "CS580_SetCurent_DC.vi"("error in"=w333, "Current (A)"=w335, "VISA Refnum in"=w334) -> ("error out"=w331:errorcluster, "VISA resource name out"=w332:refnum<visa-resource-name>)  [unwired: 7 in]
                  }
                  frame True {
                    n133 = local write "Mask"(w336) -> ()
                    n134 = call "CS580_SetCurent_DC.vi"("error in"=w341, "Current (A)"=0.001, "VISA Refnum in"=w340) -> ("error out"=w339:errorcluster, "VISA resource name out"=w338:refnum<visa-resource-name>)  [unwired: 7 in]
                  }
                }
                n135 = while {
                  shift-right: [w349] -> _
                  shift-left: w328 -> [w358]
                  tunnel: w319 -> [_]
                  tunnel: w318 -> [_]
                  stop <- w343 stop-if-true
                  n136 = Rotate 1D Array(1:w358, 2:1 ("n")) -> (0:w361:dbl[])
                  n137 = Wait (ms)(milliseconds to wait=u32 300) -> ()  [unwired: 1 out]
                  n138 = local read "Test?"() -> (w345:bool)
                  n139 = local read "T_H"() -> (w357:dbl)
                  n140 = case shown="False" w345 {
                    tunnel: [1.0 ("y") 1e-09 ("y")] -> w348
                    frame True {
                    }
                    frame False {
                    }
                  }
                  n141 = call-poly <vilib>:"Ramp Pattern.vi"("start"=1.0, "end"=100.0, "delta"=1.0) -> ("Ramp Pattern"=w352:dbl[])  [unwired: 6 in, 2 out]
                  n142 = Replace Array Subset(array=w361, new element=w357, index=0 ("Index")) -> (w349:dbl[])
                  n143 = call <vilib>:"Linear Fit.vi"("Y"=w349, "X"=w352) -> ("slope"=w351:dbl)  [unwired: 9 in, 4 out]
                  n144 = call <vilib>:"Std Deviation and Variance.vi"("X"=w349) -> ("mean"=w346:dbl)  [unwired: 1 in, 2 out]
                  n145 = Multiply(x=w346, y=w348) -> (x*y=w347:dbl)
                  n146 = Absolute Value(x=w351) -> (abs(x)=w350:dbl)
                  n147 = local read "Global Stop"() -> (w342:bool)
                  n148 = Less?(x=w350, y=w347) -> (x < y?=w344:bool)
                  n149 = Or(x=w344, y=w342) -> (x .or. y?=w343:bool)
                }
                n150 = Multiply(x=w310, y=0.8) -> (x*y=w308:dbl)
                n151 = call "setDC.vi"("VISA Refnum in"=w307, "Output Response"=KE6221_--_Output_Response."Slow", "Output State"=KE622x_--_On_Off_Control."On", "Analog Filter State"=KE622x_--_On_Off_Control."Off", "Instrument Type"=KE622x_--_Instrument_Type."KE6221", "Current Level (A)"=w308, "Voltage Limit (V)"=T3 40.0) -> ("error out"=→"error out":errorcluster)  [unwired: 6 in, 2 out]
              }
            }
            n152 = local read "Global Stop"() -> (w295:bool)
            n153 = Bundle By Name(cluster=w299, "error out"=w298) -> (w297:T7)
          }
          frame "Measure (heat)" {
            w376 = Kxx_Kxy_state_machine_cases."Turn off Heater"  # States
            # "WAIT 5 MINS, MEASURE FOR THERMAL CONDUCTIVITY"
            n154 = Unbundle By Name(w366) -> ("HTR Voltage Array"=w375:dbl[], "T_H Array"=w374:dbl[], "T_C1 Array"=w373:dbl[], "T_C2 Array"=w372:dbl[])
            n155 = local read "Calibration Only?"() -> (w377:bool)
            n156 = case shown="False" w377 {
              tunnel: w375 -> [w386 w413]
              tunnel: w374 -> [w385 w412]
              tunnel: w373 -> [w384 w411]
              tunnel: w372 -> [w383 w410]
              tunnel: [w382 w413] -> w371
              tunnel: [w381 w412] -> w370
              tunnel: [w380 w411] -> w369
              tunnel: [w379 w410] -> w368
              frame False {
                w378 = 2.0 ("Mask")
                n157 = local read "Test?"() -> (w388:bool)
                n158 = case shown="False" w388 {
                  tunnel: [300.0 3.0] -> w387
                  tunnel: w378 -> [_ _]
                  frame False {
                  }
                  frame True {
                  }
                }
                n159 = local write "Mask"(w378) -> ()
                n160 = while {
                  shift-right: [w408] -> w379
                  shift-left: w383 -> [w409]
                  shift-right: [w405] -> w381
                  shift-left: w385 -> [w406]
                  shift-right: [w402] -> w382
                  shift-left: w386 -> [w403]
                  shift-right: [w395] -> w380
                  shift-left: w384 -> [w396]
                  tunnel: w387 -> [w391]
                  i -> [w399]
                  stop <- w392 stop-if-true
                  n161 = Wait (ms)(milliseconds to wait=u32 300) -> ()  [unwired: 1 out]
                  n162 = Equal To 0?(x=w399) -> (x = 0?=w398:bool)
                  n163 = call "Elapsed Time6"("Time Target (s)"=w391, "Reset"=w398) -> ("Time has Elapsed"=w394:bool)  [unwired: 10 in, 7 out]
                  n164 = local read "HTR_Voltage"() -> (w401:dbl)
                  n165 = local read "T_C2"() -> (w407:dbl)
                  n166 = local read "T_C1"() -> (w397:dbl)
                  n167 = local read "T_H"() -> (w404:dbl)
                  n168 = Build Array (concatenate)(w403, w401) -> (w402:dbl[])
                  n169 = Build Array (concatenate)(w409, w407) -> (w408:dbl[])
                  n170 = Build Array (concatenate)(w396, w397) -> (w395:dbl[])
                  n171 = Build Array (concatenate)(w406, w404) -> (w405:dbl[])
                  n172 = local read "Global Stop"() -> (w393:bool)
                  n173 = Or(x=w394, y=w393) -> (x .or. y?=w392:bool)
                }
              }
              frame True {
              }
            }
            n174 = local read "Global Stop"() -> (w364:bool)
            n175 = Bundle By Name(cluster=w366, "HTR Voltage Array"=w371, "T_H Array"=w370, "T_C1 Array"=w369, "T_C2 Array"=w368) -> (w367:T7)
          }
          frame "Turn off Heater" {
            w430 = Kxx_Kxy_state_machine_cases."Assign Heater Current"  # States
            # "FIGURE OUT NEW HEATER CURRENT"
            n176 = local read "Calibration Only?"() -> (w432:bool)
            n177 = Unbundle By Name(w425) -> ("HTR Voltage Array"=w429:dbl[], "T_H Array"=w426:dbl[], "T_C1 Array"=w427:dbl[], "T_C2 Array"=w428:dbl[], "error out"=w424:errorcluster)
            n178 = case shown="False" w432 {
              tunnel: w431 -> [w448 w469]
              tunnel: w424 -> [w447 w468]
              tunnel: w428 -> [w437 w459]
              tunnel: w426 -> [w438 w460]
              tunnel: w429 -> [w439 w461]
              tunnel: [w455 w477] -> w421
              tunnel: [w440 w464] -> w422
              tunnel: [w449 w471] -> w419
              tunnel: [w446 w467] -> w423
              tunnel: w427 -> [w436 w458]
              tunnel: [w442 w466] -> w420
              tunnel: 2.5 ("Mask") -> [w435 w457]
              tunnel: w414 -> [w434 _]
              frame False {
                n179 = local write "Mask"(w435) -> ()
                n180 = call-poly <vilib>:"Mean.vi"("X"=w439) -> ("mean"=w453:dbl)  [unwired: 1 out]
                n181 = call-poly <vilib>:"Mean.vi"("X"=w437) -> ("mean"=w444:dbl)  [unwired: 1 out]
                n182 = local read "HTR_Current"() -> (w454:dbl)
                n183 = VISA Write(VISA resource name=w448, write buffer="SOUT 0", error in (no error)=w447) -> (error out=w446:errorcluster)  [unwired: 2 out]
                n184 = call-poly <vilib>:"Mean.vi"("X"=w436) -> ("mean"=w443:dbl)  [unwired: 1 out]
                n185 = call-poly <vilib>:"Mean.vi"("X"=w438) -> ("mean"=w452:dbl)  [unwired: 1 out]
                n186 = Multiply(x=w454, y=w453) -> (x*y=w441:dbl)
                n187 = Subtract(x=w444, y=w443) -> (x-y=w442:dbl)
                n188 = Subtract(x=w452, y=w444) -> (x-y=w455:dbl)
                n189 = call "KE622x -- Set Output State.vi"("Resource In"=w434, "Output State"=KE622x_--_On_Off_Control."Off") -> ()  [unwired: 12 in, 2 out]
                n190 = Add(x=w452, y=w444) -> (x+y=w451:dbl)
                n191 = Absolute Value(x=w441) -> (abs(x)=w440:dbl)
                n192 = Divide(x=w451, y=2.0) -> (x/y=w449:dbl)
                n193 = Wait (ms)(milliseconds to wait=u32 5000) -> ()  [unwired: 1 out]
              }
              frame True {
                n194 = call-poly <vilib>:"Mean.vi"("X"=w461) -> ("mean"=w475:dbl)  [unwired: 1 out]
                n195 = call-poly <vilib>:"Mean.vi"("X"=w458) -> ("mean"=w463:dbl)  [unwired: 1 out]
                n196 = call-poly <vilib>:"Mean.vi"("X"=w460) -> ("mean"=w474:dbl)  [unwired: 1 out]
                n197 = call-poly <vilib>:"Mean.vi"("X"=w459) -> ("mean"=w462:dbl)  [unwired: 1 out]
                n198 = local write "Mask"(w457) -> ()
                n199 = Wait (ms)(milliseconds to wait=u32 5000) -> ()  [unwired: 1 out]
                n200 = Subtract(x=w462, y=w463) -> (x-y=w466:dbl)
                n201 = Subtract(x=w474, y=w462) -> (x-y=w477:dbl)
                n202 = Add(x=w474, y=w462) -> (x+y=w473:dbl)
                n203 = VISA Write(VISA resource name=w469, write buffer="SOUT 0", error in (no error)=w468) -> (error out=w467:errorcluster)  [unwired: 2 out]
                n204 = local read "HTR_Current"() -> (w476:dbl)
                n205 = Divide(x=w473, y=2.0) -> (x/y=w471:dbl)
                n206 = Multiply(x=w476, y=w475) -> (x*y=w465:dbl)
                n207 = Absolute Value(x=w465) -> (abs(x)=w464:dbl)
              }
            }
            n208 = Bundle By Name(cluster=w425, "T_avg"=w419, "dTxx"=w421, "dTxy"=w420, "HTR Power"=w422, "error out"=w423) -> (w418:T7)
            n209 = local read "Global Stop"() -> (w416:bool)
          }
          frame "Assign Heater Current" {
            w484 = Kxx_Kxy_state_machine_cases."Plot Kxx, Kxy"  # States
            n210 = local read "Preset Heater Current Array?"() -> (w485:bool)
            n211 = Unbundle By Name(w482) -> ("dTxx"=w483:dbl)
            n212 = case shown="False" w485 {
              tunnel: w483 -> [w491 _]
              tunnel: w480 -> [_ w504]
              frame False {
                n213 = local read "DeltaT (fraction of tsp)"() -> (w486:dbl)
                n214 = local read "Tsp"() -> (w493:dbl)
                n215 = Multiply(x=w486, y=w493) -> (x*y=w492:dbl)
                n216 = Divide(x=w492, y=w491) -> (x/y=w490:dbl)
                n217 = Square Root(x=w490) -> (sqrt(x)=w489:dbl)
                n218 = Less?(x=w489, y=1.6) -> (x < y?=w487:bool)
                n219 = case shown="True" w487 {
                  tunnel: w489 -> [_ w501]
                  frame False {
                    n220 = local read "HTR_Current"() -> (w495:dbl)
                    n221 = Multiply(x=w495, y=1.3) -> (x*y=w494:dbl)
                    n222 = local write "HTR_Current"(w494) -> ()
                  }
                  frame True {
                    n223 = local read "HTR_Current"() -> (w500:dbl)
                    n224 = Multiply(x=w500, y=w501) -> (x*y=w498:dbl)
                    n225 = Less?(x=w498, y=0.00075) -> (x < y?=w497:bool)
                    n226 = case shown="True" w497 {
                      tunnel: w498 -> [_ w503]
                      frame False {
                        n227 = local write "HTR_Current"(0.00075 ("HTR_Current")) -> ()
                      }
                      frame True {
                        n228 = local write "HTR_Current"(w503) -> ()
                      }
                    }
                  }
                }
              }
              frame True {
                n229 = local write "HTR_Current"(w504) -> ()
              }
            }
            n230 = local read "Global Stop"() -> (w479:bool)
          }
          frame "Plot Kxx, Kxy" {
            w522 = Kxx_Kxy_state_machine_cases."End"  # States
            n231 = local read "Sample_w"() -> (w518:dbl)
            n232 = local read "Sample_Lxx"() -> (w516:dbl)
            n233 = local read "Sample_t"() -> (w517:dbl)
            n234 = local read "Sample_Lxy"() -> (w527:dbl)
            n235 = Unbundle By Name(w521) -> ("T_avg"=w520:dbl, "dTxx"=w519:dbl, "dTxy"=w507:dbl, "HTR Power"=w506:dbl)
            n236 = call "Kxx_Kxy_calc.vi"("Sample_w"=w518, "HTR Power"=w506, "Sample_t"=w517, "dTxy"=w507, "dTxx"=w519, "Sample_Lxx"=w516, "Sample_Lxy"=w527) -> ("Kxx"=w526:dbl, "Kxy"=w525:dbl)  [unwired: 3 in]
            n237 = Unbundle By Name(w512) -> ("T_avg data"=w515:dbl[], "Kxx data"=w514:dbl[], "Kxy data"=w513:dbl[])
            n238 = Build Array (concatenate)(w514, w526) -> (w510:dbl[])
            n239 = Build Array (concatenate)(w513, w525) -> (w509:dbl[])
            n240 = Build Array (concatenate)(w515, w520) -> (w511:dbl[])
            n241 = local read "Calibration Only?"() -> (w523:bool)
            n242 = Bundle(w511, w509) -> (w524:cluster{dbl[], dbl[]})  [unwired: 1 in]
            n243 = Bundle(w511, w510) -> (w528:cluster{dbl[], dbl[]})  [unwired: 1 in]
            n244 = case shown="False" w523 {
              tunnel: w528 -> [_ w530]
              tunnel: w524 -> [_ w529]
              frame True {
              }
              frame False {
                "Kxx Plot" <- w530
                "Kxy Plot" <- w529
              }
            }
            n245 = Bundle By Name(cluster=w512, "T_avg data"=w511, "Kxx data"=w510, "Kxy data"=w509) -> (w508:T6)
            n246 = local read "Global Stop"() -> (w505:bool)
          }
          frame "End" {
          }
        }
        n247 = Wait (ms)(milliseconds to wait=u32 10) -> ()  [unwired: 1 out]
      }
      n248 = local read "Global Stop"() -> (w169:bool)
    }
    n249 = local read "Global Stop"() -> (w144:bool)
    "Fieldsp" <- w164
  }
  n250 = property on="Field selection" class="Ring (strict)"("Strings []"=w62) -> ()  [unwired: 2 in, 2 out]
  n251 = property on="Name" class="Ring (strict)"("Strings []"=w3) -> ()  [unwired: 2 in, 2 out]
  n252 = Tick Count (ms)() -> (millisecond timer value=w38:u32)
  n253 = while {
    tunnel: w38 -> [w587]
    shift-right: [w581] -> _
    shift-left: 0 -> [w586]
    tunnel: w3 -> [w582]
    shift-right: [w577] -> _
    shift-left: dbl[][] [] -> [w578]
    tunnel: "Delay (ms)" -> [w571]
    tunnel: w50 -> [w563]
    tunnel: [w537] -> w25
    shift-right: [w536] -> w15
    shift-left: w49 -> [w560]
    stop <- "Finish" stop-if-true
    # "PLOT DATA BEING RECORDED TO FILE CONTINUOUSLY"
    n254 = Wait (ms)(milliseconds to wait=w571) -> ()  [unwired: 1 out]
    n255 = Tick Count (ms)() -> (millisecond timer value=w588:u32)
    n256 = local read "T_C1 Lockin"() -> (w546:enum16{"LI1", "LI2", "LI3"})
    n257 = local read "T_C2 Lockin"() -> (w545:enum16{"LI1", "LI2", "LI3"})
    n258 = local read "T_H Lockin"() -> (w547:enum16{"LI1", "LI2", "LI3"})
    n259 = global read "MQM Data Transfer All.vi" "ZI MFLI"() -> (w539:T8)
    n260 = VISA Write(VISA resource name=w563, write buffer="FETC?", error in (no error)=w560) -> (VISA resource name out=w562:refnum<visa-resource-name>, error out=w559:errorcluster)  [unwired: 1 out]
    n261 = Subtract(x=w588, y=w587) -> (x-y=w581:u32)
    n262 = case shown="\"LI1\", Default" w547 {
      tunnel: w539 -> [w609 w612 w615]
      tunnel: [w608 w611 w614] -> w549
      tunnel: [w607 w610 w613] -> w548
      frame "LI1", Default {
        n263 = Unbundle By Name(w609) -> ("Lockin 1 Demod 0.X(V)"=w608:dbl, "Lockin 1 Demod 0.Theta (deg)"=w607:dbl)
      }
      frame "LI2" {
        n264 = Unbundle By Name(w612) -> ("Lockin 2 Demod 0.X(V)"=w611:dbl, "Lockin 2 Demod 0.Theta (deg)"=w610:dbl)
      }
      frame "LI3" {
        n265 = Unbundle By Name(w615) -> ("Lockin 3 Demod 0.X(V)"=w614:dbl, "Lockin 3 Demod 0.Theta (deg)"=w613:dbl)
      }
    }
    n266 = case shown="\"LI2\", Default" w546 {
      tunnel: [w598 w603 w604] -> w574
      tunnel: [w599 w602 w605] -> w553
      tunnel: w539 -> [w600 w601 w606]
      frame "LI1" {
        n267 = Unbundle By Name(w600) -> ("Lockin 1 Demod 0.X(V)"=w599:dbl, "Lockin 1 Demod 0.Theta (deg)"=w598:dbl)
      }
      frame "LI2", Default {
        n268 = Unbundle By Name(w601) -> ("Lockin 2 Demod 0.X(V)"=w602:dbl, "Lockin 2 Demod 0.Theta (deg)"=w603:dbl)
      }
      frame "LI3" {
        n269 = Unbundle By Name(w606) -> ("Lockin 3 Demod 0.X(V)"=w605:dbl, "Lockin 3 Demod 0.Theta (deg)"=w604:dbl)
      }
    }
    n270 = case shown="\"LI3\", Default" w545 {
      tunnel: [w589 w594 w595] -> w542
      tunnel: [w590 w593 w596] -> w543
      tunnel: w539 -> [w591 w592 w597]
      frame "LI1" {
        n271 = Unbundle By Name(w591) -> ("Lockin 1 Demod 0.X(V)"=w590:dbl, "Lockin 1 Demod 0.Theta (deg)"=w589:dbl)
      }
      frame "LI2" {
        n272 = Unbundle By Name(w592) -> ("Lockin 2 Demod 0.X(V)"=w593:dbl, "Lockin 2 Demod 0.Theta (deg)"=w594:dbl)
      }
      frame "LI3", Default {
        n273 = Unbundle By Name(w597) -> ("Lockin 3 Demod 0.X(V)"=w596:dbl, "Lockin 3 Demod 0.Theta (deg)"=w595:dbl)
      }
    }
    n274 = global read "MQM Data Transfer All.vi" "PPMS"() -> (w538:T9)
    n275 = Subtract(x=w581, y=w586) -> (x-y=→"Data Rate (ms)":u32)
    n276 = Unbundle By Name(w538) -> ("Temperature.Temperature (K)"=w580:dbl, "Field.Field (T)"=w579:dbl)
    n277 = VISA Read(VISA resource name=w562, byte count=u32 1000, error in (no error)=w559) -> (VISA resource name out=w537:refnum<visa-resource-name>, read buffer=w558:string, error out=w536:errorcluster)  [unwired: 1 out]
    n278 = Build Array(w581, w580, w579) -> (w575:dbl[])
    n279 = Match Pattern(string=w558, regular expression="VDC", offset (0)=0) -> (before substring=w555:string)  [unwired: 3 out]
    n280 = Build Array (concatenate)(w575, w549, w548) -> (w573:dbl[])
    n281 = Fract/Exp String To Number(string=w555) -> (number=w554:dbl)  [unwired: 3 in, 1 out]
    n282 = Build Array (concatenate)(w573, w553, w574) -> (w544:dbl[])
    n283 = local read "HTR_Voltage"() -> (w566:dbl)
    n284 = local read "HTR_Current"() -> (w570:dbl)
    n285 = local read "I_therm"() -> (w552:dbl)
    n286 = local read "Fieldsp"() -> (w535:dbl)
    n287 = local write "HTR_Voltage"(w554) -> ()
    n288 = Build Array (concatenate)(w544, w543, w542) -> (w541:dbl[])
    n289 = local read "Mask"() -> (w568:dbl)
    n290 = local read "T_C1"() -> (w551:dbl)
    n291 = local read "T_C2"() -> (w550:dbl)
    n292 = local read "T_H"() -> (w540:dbl)
    n293 = local read "Tsp"() -> (w567:dbl)
    n294 = Build Array (concatenate)(w541, w566, w570, w568, w567, w552, w540, w551, w550, w535) -> (w569:dbl[])
    n295 = Build Array (concatenate)(w578, w569) -> (w572:dbl[][])
    n296 = flat-sequence {
      tunnel: "Display Elements" -> [w628]
      tunnel: [w621] -> w585
      tunnel: w582 -> [w617]
      tunnel: w572 -> [w616]
      tunnel: w585 -> [w675]
      frame #0 {
        n297 = for {
          tunnel: w628 -> [w657] mode=indexing
          shift-right: [w649] -> w627
          shift-left: dbl[] [] -> [w648]
          shift-right: [w650] -> w625
          shift-left: dbl[][] [] -> [w659]
          shift-right: [w655] -> w621
          shift-left: string[] [] -> [w654]
          tunnel: w617 -> [w651]
          tunnel: w616 -> [w652]
          i -> [w653]
          n298 = Unbundle By Name(w657) -> ("X"=w658:bool, "Y"=w661:bool, "Name"=w656:u16)
          n299 = Index Array(array=w652, index (col)=w656) -> (element=w660:dbl[])  [unwired: 1 in]
          n300 = case shown="False" w661 {
            tunnel: w660 -> [_ w667]
            tunnel: w659 -> [w665 w674]
            tunnel: [w665 w673] -> w650
            tunnel: w656 -> [_ w672]
            tunnel: [w666 w670] -> w655
            tunnel: w654 -> [w666 w669]
            tunnel: w651 -> [_ w668]
            frame False {
            }
            frame True {
              n301 = Build Array (concatenate)(w674, w667) -> (w673:dbl[][])
              n302 = Index Array(array=w668, index=w672) -> (element=w671:string)
              n303 = Build Array (concatenate)(w669, w671) -> (w670:string[])
            }
          }
          n304 = case shown="False" w658 {
            tunnel: w656 -> [_ w664]
            tunnel: w653 -> [_ _]
            tunnel: w651 -> [_ w662]
            frame False {
            }
            frame True {
              n305 = Index Array(array=w662, index=w664) -> (element=w663:string)
              n306 = property on="All Data" class="XYGraph (strict)"("XScale.NameLbl.Text"=w663) -> ()  [unwired: 2 in, 2 out]
            }
          }
          n307 = Select(t=w660, s=w658, f=w648) -> (s? t:f=w649:dbl[])
        }
        n308 = for {
          tunnel: w625 -> [w632] mode=indexing
          tunnel: w627 -> [w634]
          tunnel: [w635] -> w626 mode=indexing
          n309 = case shown="0, Default" "Y-Axis" {
            tunnel: w632 -> [w636 w638 w641]
            tunnel: [w636 w637 w640] -> w629
            frame 0, Default {
            }
            frame 1 {
              n310 = Reciprocal(x=w638) -> (1/x=w637:dbl[])
            }
            frame 2 {
              n311 = Absolute Value(x=w641) -> (abs(x)=w639:dbl[])
              n312 = Logarithm Base 10(1:w639) -> (0:w640:dbl[])
            }
          }
          n313 = case shown="0, Default" "X-Axis" {
            tunnel: w634 -> [w642 w644 w647]
            tunnel: [w642 w643 w646] -> w633
            frame 0, Default {
            }
            frame 1 {
              n314 = Reciprocal(x=w644) -> (1/x=w643:dbl[])
            }
            frame 2 {
              n315 = Absolute Value(x=w647) -> (abs(x)=w645:dbl[])
              n316 = Logarithm Base 10(1:w645) -> (0:w646:dbl[])
            }
          }
          n317 = Bundle(w633, w629) -> (w635:cluster{dbl[], dbl[]})  [unwired: 1 in]
        }
        "All Data" <- w626
        n318 = Array Size(array=w625) -> (size(s)=w624:i32[])
        n319 = Index Array(array=w624, index=0) -> (element=w622:i32)
        n320 = property on="All Data" class="XYGraph (strict)"("LegNumRows"=w622) -> ()  [unwired: 2 in, 2 out]
      }
      frame #1 {
        n321 = for {
          tunnel: w675 -> [w676] mode=indexing
          i -> [w677]
          n322 = property on="All Data" class="XYGraph (strict)"("Active Plot"=w677, "Plot.Plot Name"=w676) -> ()  [unwired: 2 in, 2 out]
        }
      }
    }
    n323 = call "Data length guard.vi"("Max length"=20000, "Array"=w572) -> ("array w/ subset deleted"=w577:dbl[][])  [unwired: 9 in]
    "Global Stop" <- "Finish"
  }
  n324 = case shown="True" "Quick Data Recording" {
    tunnel: w37 -> [_ w681]
    tunnel: "Delay (ms)" -> [_ w679]
    tunnel: w3 -> [_ w678]
    frame False {
    }
    frame True {
      # "SAVE DATA TO FILE"
      n325 = Strip Path(path=w681) -> (stripped path=w685:path, name=w682:string)
      n326 = Concatenate Strings(w682, ".dat") -> (w684:string)
      n327 = Tick Count (ms)() -> (millisecond timer value=w688:u32)
      n328 = Build Path(base path=w685, name or relative path=w684) -> (appended path=w686:path)
      n329 = call-poly <vilib>:"Write To Spreadsheet File.vi"("append to file? (new file:F)"=TRUE, "1D data"=w678, "file path (dialog if empty)"=w686) -> ("new file path (Not A Path if cancelled)"=w680:path)  [unwired: 5 in]
      n330 = while {
        tunnel: w688 -> [w716]
        tunnel: w680 -> [w708]
        tunnel: w679 -> [w707]
        stop <- w689 stop-if-true
        n331 = Wait (ms)(milliseconds to wait=w707) -> ()  [unwired: 1 out]
        n332 = Tick Count (ms)() -> (millisecond timer value=w715:u32)
        n333 = local read "T_C1 Lockin"() -> (w704:enum16{"LI1", "LI2", "LI3"})
        n334 = local read "T_C2 Lockin"() -> (w699:enum16{"LI1", "LI2", "LI3"})
        n335 = local read "T_H Lockin"() -> (w705:enum16{"LI1", "LI2", "LI3"})
        n336 = global read "MQM Data Transfer All.vi" "ZI MFLI"() -> (w691:T8)
        n337 = Subtract(x=w715, y=w716) -> (x-y=w714:u32)
        n338 = case shown="\"LI1\", Default" w705 {
          tunnel: w691 -> [w737 w740 w743]
          tunnel: [w736 w739 w742] -> w703
          tunnel: [w735 w738 w741] -> w702
          frame "LI1", Default {
            n339 = Unbundle By Name(w737) -> ("Lockin 1 Demod 0.X(V)"=w736:dbl, "Lockin 1 Demod 0.Theta (deg)"=w735:dbl)
          }
          frame "LI2" {
            n340 = Unbundle By Name(w740) -> ("Lockin 2 Demod 0.X(V)"=w739:dbl, "Lockin 2 Demod 0.Theta (deg)"=w738:dbl)
          }
          frame "LI3" {
            n341 = Unbundle By Name(w743) -> ("Lockin 3 Demod 0.X(V)"=w742:dbl, "Lockin 3 Demod 0.Theta (deg)"=w741:dbl)
          }
        }
        n342 = case shown="\"LI2\", Default" w704 {
          tunnel: w691 -> [w726 w731 w734]
          tunnel: [w728 w730 w733] -> w701
          tunnel: [w727 w729 w732] -> w700
          frame "LI1" {
            n343 = Unbundle By Name(w726) -> ("Lockin 1 Demod 0.X(V)"=w728:dbl, "Lockin 1 Demod 0.Theta (deg)"=w727:dbl)
          }
          frame "LI2", Default {
            n344 = Unbundle By Name(w731) -> ("Lockin 2 Demod 0.X(V)"=w730:dbl, "Lockin 2 Demod 0.Theta (deg)"=w729:dbl)
          }
          frame "LI3" {
            n345 = Unbundle By Name(w734) -> ("Lockin 3 Demod 0.X(V)"=w733:dbl, "Lockin 3 Demod 0.Theta (deg)"=w732:dbl)
          }
        }
        n346 = case shown="\"LI3\", Default" w699 {
          tunnel: w691 -> [w717 w722 w725]
          tunnel: [w719 w721 w724] -> w698
          tunnel: [w718 w720 w723] -> w697
          frame "LI1" {
            n347 = Unbundle By Name(w717) -> ("Lockin 1 Demod 0.X(V)"=w719:dbl, "Lockin 1 Demod 0.Theta (deg)"=w718:dbl)
          }
          frame "LI2" {
            n348 = Unbundle By Name(w722) -> ("Lockin 2 Demod 0.X(V)"=w721:dbl, "Lockin 2 Demod 0.Theta (deg)"=w720:dbl)
          }
          frame "LI3", Default {
            n349 = Unbundle By Name(w725) -> ("Lockin 3 Demod 0.X(V)"=w724:dbl, "Lockin 3 Demod 0.Theta (deg)"=w723:dbl)
          }
        }
        n350 = global read "MQM Data Transfer All.vi" "PPMS"() -> (w690:T9)
        n351 = Unbundle By Name(w690) -> ("Temperature.Temperature (K)"=w713:dbl, "Field.Field (T)"=w712:dbl)
        n352 = local read "HTR_Voltage"() -> (w696:dbl)
        n353 = local read "HTR_Current"() -> (w695:dbl)
        n354 = local read "I_therm"() -> (w692:dbl)
        n355 = local read "Mask"() -> (w694:dbl)
        n356 = local read "Tsp"() -> (w693:dbl)
        n357 = Build Array(w714, w713, w712, w703, w702, w701, w700, w698, w697, w696, w695, w694, w693, w692) -> (w711:dbl[])
        n358 = call "Write To Spreadsheet File (DBL)2.vi"("format (%.3f)"="%_8f", "append to file? (new file:F)"=TRUE, "1D data"=w711, "file path (dialog if empty)"=w708) -> ("error out"=w706:errorcluster)  [unwired: 3 in, 1 out]
        n359 = local read "Global Stop"() -> (w689:bool)
        n360 = call <vilib>:"Clear Errors.vi"("error in (no error)"=w706) -> ()  [unwired: 5 in, 2 out]
      }
    }
  }
  n361 = while {
    tunnel: "Delay (ms)" -> [w765]
    tunnel: w3 -> [_]
    stop <- w745 stop-if-true
    # "CONVERT RESISTANCE TO TEMPERATURE"
    n362 = global read "MQM Data Transfer All.vi" "ZI MFLI"() -> (w744:T8)
    n363 = Wait (ms)(milliseconds to wait=w765) -> ()  [unwired: 1 out]
    n364 = local read "T_C2 Lockin"() -> (w752:enum16{"LI1", "LI2", "LI3"})
    n365 = local read "T_C1 Lockin"() -> (w758:enum16{"LI1", "LI2", "LI3"})
    n366 = local read "T_H Lockin"() -> (w759:enum16{"LI1", "LI2", "LI3"})
    n367 = local read "I_therm"() -> (w761:dbl)
    n368 = case shown="\"LI3\", Default" w752 {
      tunnel: w744 -> [w767 w768 w771]
      tunnel: [w766 w769 w770] -> w754
      frame "LI1" {
        n369 = Unbundle By Name(w767) -> ("Lockin 1 Demod 0.X(V)"=w766:dbl)
      }
      frame "LI2" {
        n370 = Unbundle By Name(w768) -> ("Lockin 2 Demod 0.X(V)"=w769:dbl)
      }
      frame "LI3", Default {
        n371 = Unbundle By Name(w771) -> ("Lockin 3 Demod 0.X(V)"=w770:dbl)
      }
    }
    n372 = case shown="\"LI1\", Default" w759 {
      tunnel: w744 -> [w779 w780 w783]
      tunnel: [w778 w781 w782] -> w757
      frame "LI1", Default {
        n373 = Unbundle By Name(w779) -> ("Lockin 1 Demod 0.X(V)"=w778:dbl)
      }
      frame "LI2" {
        n374 = Unbundle By Name(w780) -> ("Lockin 2 Demod 0.X(V)"=w781:dbl)
      }
      frame "LI3" {
        n375 = Unbundle By Name(w783) -> ("Lockin 3 Demod 0.X(V)"=w782:dbl)
      }
    }
    n376 = case shown="\"LI2\", Default" w758 {
      tunnel: w744 -> [w773 w775 w777]
      tunnel: [w772 w774 w776] -> w756
      frame "LI1" {
        n377 = Unbundle By Name(w773) -> ("Lockin 1 Demod 0.X(V)"=w772:dbl)
      }
      frame "LI2", Default {
        n378 = Unbundle By Name(w775) -> ("Lockin 2 Demod 0.X(V)"=w774:dbl)
      }
      frame "LI3" {
        n379 = Unbundle By Name(w777) -> ("Lockin 3 Demod 0.X(V)"=w776:dbl)
      }
    }
    n380 = local read "R_C2 Log Domain"() -> (w751:dbl[])
    n381 = local read "R_C1 Log Domain"() -> (w747:dbl[])
    n382 = local read "R_H Log Domain"() -> (w749:dbl[])
    n383 = Square Root(x=2.0) -> (sqrt(x)=w763:dbl)
    n384 = local read "R_C2 coeffs"() -> (w750:dbl[])
    n385 = local read "R_C1 coeffs"() -> (w746:dbl[])
    n386 = local read "R_H coeffs"() -> (w748:dbl[])
    n387 = Divide(x=w761, y=w763) -> (x/y=w753:dbl)
    n388 = call "cheby6.vi"("I"=w753, "Coefs"=w750, "RU/L"=w751, "LIX"=w754) -> ("T"=w755:dbl)
    n389 = call "cheby6.vi"("I"=w753, "Coefs"=w748, "RU/L"=w749, "LIX"=w757) -> ("T"=w760:dbl)
    n390 = call "cheby6.vi"("I"=w753, "Coefs"=w746, "RU/L"=w747, "LIX"=w756) -> ("T"=w764:dbl)
    n391 = local read "Global Stop"() -> (w745:bool)
    n392 = local write "T_C2"(w755) -> ()
    n393 = local write "T_C1"(w764) -> ()
    n394 = local write "T_H"(w760) -> ()
  }
  n395 = Unbundle By Name(w24) -> ("error out"=w23:errorcluster)
  n396 = VISA Close(VISA resource name=w4) -> ()  [unwired: 1 in, 1 out]
  n397 = VISA Close(VISA resource name=w20, error in (no error)=w17) -> (error out=→"KE6221 error out":errorcluster)
  n398 = call <instrlib>:"SetTemperature.vi"("Rate"=3.0, "Temperature"="Final Temperature (K)", "error in (no error)"=w23, "Instrument Ref In"=w21) -> ("error out"=w44:errorcluster, "Instrument Ref Out"=w45:refnum<k24>)  [unwired: 3 in, 1 out]
  n399 = call <instrlib>:"SetField.vi"("Rate"=100.0, "Field"="Final Field (Oe)", "error in (no error)"=w44, "Instrument Ref In"=w45) -> ("error out"=→"QD error out":errorcluster)  [unwired: 3 in, 2 out]
  n400 = VISA Close(VISA resource name=w25, error in (no error)=w15) -> (error out=→"KE2182 error out":errorcluster)
